vi "ASDA-A2_Get Servo Status.vi"(8 "error in":errorcluster, 11 "Buffer Data In":T2) -> (0 "error out":errorcluster, 2 "Sevro Status":T1, 3 "Buffer Data Out":T2)   [LabVIEW 2016]
uses:
  Data Def/ASDA-A2_Buffer Data.ctl
  Data Def/ASDA-A2_Read Register Data.ctl
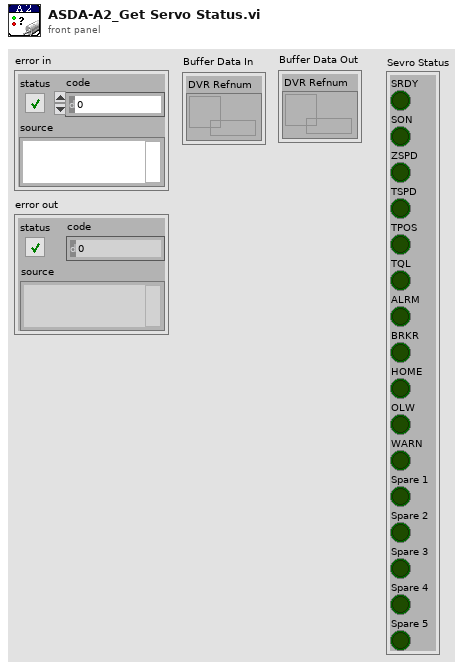
[diagram p1: front panel]
types:
  T1 = cluster{"SRDY":bool, "SON":bool, "ZSPD":bool, "TSPD":bool, "TPOS":bool, "TQL":bool, "ALRM":bool, "BRKR":bool, "HOME":bool, "OLW":bool, "WARN":bool, "Spare 1":bool, "Spare 2":bool, "Spare 3":bool, "Spare 4":bool, "Spare 5":bool}
  T2 = typedef "ASDA-A2_Buffer Data.ctl" = cluster{"DVR Refnum":refnum<data-value>}
  T3 = typedef "ASDA-A2_Read Register Data.ctl" = cluster{"Address":u16, "Count":u16, "Page":string, "Description":string}
  T4 = cluster{"Boolean array[0]":bool, "Boolean array[1]":bool, "Boolean array[2]":bool, "Boolean array[3]":bool, "Boolean array[4]":bool, "Boolean array[5]":bool, "Boolean array[6]":bool, "Boolean array[7]":bool, "Boolean array[8]":bool, "Boolean array[9]":bool, "Boolean array[10]":bool, "Boolean array[11]":bool, "Boolean array[12]":bool, "Boolean array[13]":bool, "Boolean array[14]":bool, "Boolean array[15]":bool}
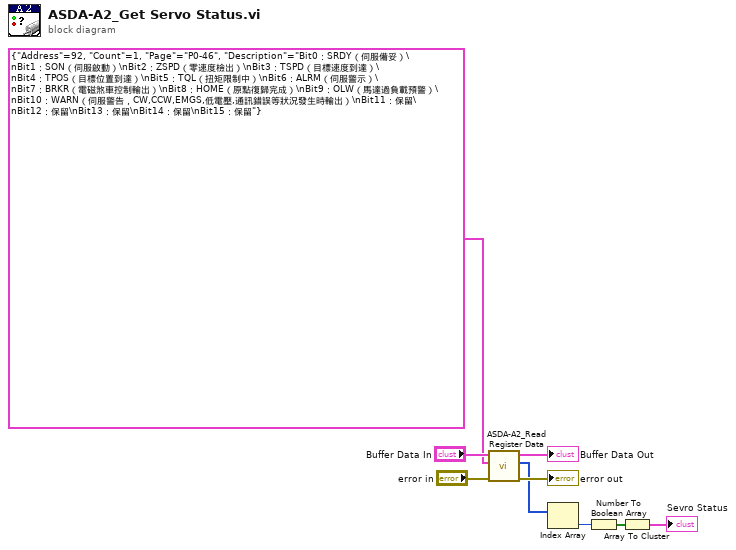
[diagram p0: block diagram]
diagram:
  n1 = call "ASDA-A2_Read Register Data.vi"("error in"="error in", "Read Register Data"=T3 {"Address"=92, "Count"=1, "Page"="P0-46", "Description"="Bit0：SRDY（伺服備妥）\nBit1：SON（伺服啟動）\nBit2：ZSPD（零速度檢出）\nBit3：TSPD（目標速度到達）\nBit4：TPOS（目標位置到達）\nBit5：TQL（扭矩限制中）\nBit6：ALRM（伺服警示）\nBit7：BRKR（電磁煞車控制輸出）\nBit8：HOME（原點復歸完成）\nBit9：OLW（馬達過負載預警）\nBit10：WARN（伺服警告，CW,CCW,EMGS,低電壓,通訊錯誤等狀況發生時輸出）\nBit11：保留\nBit12：保留\nBit13：保留\nBit14：保留\nBit15：保留"}, "Buffer Data In"="Buffer Data In") -> ("error out"=→"error out":errorcluster, "Data"=w3:u16[], "Buffer Data Out"=→"Buffer Data Out":T2)  [unwired: 6 in]
  n2 = Index Array(array=w3) -> (element=w1:u16)  [unwired: 1 in]
  n3 = Number To Boolean Array(number=w1) -> (Boolean array=w2:bool[])
  n4 = Array To Cluster(array=w2) -> (cluster=→"Sevro Status":T4)
